vi "ColorRamp.vi"(1 "Slide":dbl(slide)=10.105263157894736 scale=0.0..30.0) -> (0 "Color":u32(colorbox)=11793673)   [LabVIEW 2022 SP3]
panel:
  in  "Color Array":cluster{"Value":dbl, "Color":u32}[](array[cluster])=[{"Value"=5.0, "Color"=6618880}, {"Value"=15.0, "Color"=16771858}, {"Value"=25.0, "Color"=16711680}]
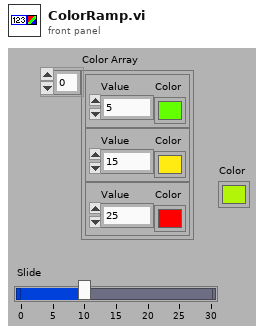
[diagram p1: front panel]
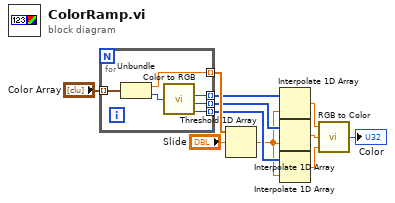
[diagram p0: block diagram]
diagram:
  n1 = for {
    tunnel: "Color Array" -> [w17] mode=indexing
    tunnel: [w15] -> w10 mode=indexing
    tunnel: [w14] -> w9 mode=indexing
    tunnel: [w13] -> w8 mode=indexing
    tunnel: [w12] -> w11 mode=indexing
    n2 = Unbundle(w17) -> ("Value"=w12:dbl, "Color"=w16:u32)
    n3 = call <vilib>:"Color to RGB.vi"("Color"=w16) -> ("R"=w15:u8, "G"=w14:u8, "B"=w13:u8)  [unwired: 1 out]
  }
  n4 = Threshold 1D Array(2:"Slide", 3:w11) -> (0:w7:dbl)  [unwired: 1 in]
  n5 = Interpolate 1D Array(1:w7, 2:w10) -> (0:w4:dbl)
  n6 = Interpolate 1D Array(1:w7, 2:w9) -> (0:w5:dbl)
  n7 = Interpolate 1D Array(1:w7, 2:w8) -> (0:w6:dbl)
  n8 = call <vilib>:"RGB to Color.vi"("B"=w6, "G"=w5, "R"=w4) -> ("Color"=→"Color":u32)
